vi "PopulateTreeSumary.vi"(8 "error in":errorcluster, 10 "array":T1[](array[typedef]), 11 "tree ref in":refnum<vi>) -> (0 "error out":errorcluster)   [LabVIEW 2013, in "NISE_CEF_TreeControl.lvlib"]
doc: "This VI will populate the tree control with the summary from the nodes. Use this when adding new nodes to tree"
uses:
  NISE_CEF_TreeControl.lvlib
  Node/Summary.ctl
  Node/NISE_CEF_Node.lvclass
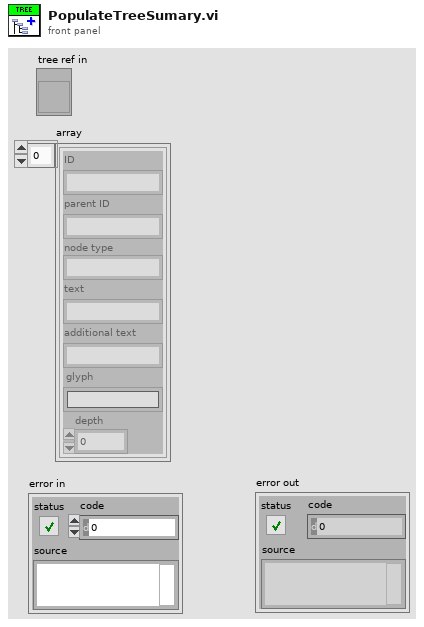
[diagram p1: front panel]
types:
  T1 = typedef "NISE_CEF_Node.lvclass/Summary.ctl" = cluster{"ID":string, "parent ID":string, "node type":string, "text":string, "additional text":string, "glyph":string, "depth":i32}
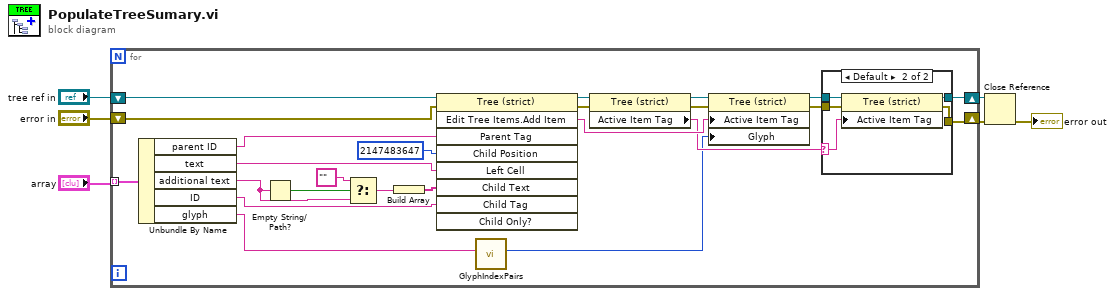
[diagram p0: block diagram]
diagram:
  n1 = for {
    tunnel: "array" -> [w15] mode=indexing
    shift-right: [w11] -> w5
    shift-left: "tree ref in" -> [w14]
    shift-right: [w9] -> w2
    shift-left: "error in" -> [w10]
    n2 = Unbundle By Name(w15) -> ("parent ID"=w30:string, "text"=w16:string, "additional text"=w8:string, "ID"=w27:string, "glyph"=w13:string)
    n3 = Empty String/Path?(string/path=w8) -> (empty?=w7:bool)
    n4 = Select(t="", s=w7, f=w8) -> (s? t:f=w25:string)
    n5 = Build Array(w25) -> (w28:string[])
    n6 = invoke class="Tree (strict)" method="Edit Tree Items.Add Item"(reference=w14, error in=w10, "Parent Tag"=w30, "Child Position"=2147483647 ("child Position"), "Left Cell"=w16, "Child Text"=w28, "Child Tag"=w27) -> (reference out=w24:refnum<vi>, error out=w23:errorcluster, "Edit Tree Items:Add Item"=w20:string)  [unwired: 2 in, 6 out]
    n7 = call "GlyphIndexPairs.vi"("glyph"=w13) -> ("index"=w12:i32)  [unwired: 10 in]
    n8 = property class="Tree (strict)"(reference=w24, error in=w23) -> (reference out=w22:refnum<vi>, error out=w21:errorcluster, "Active Item Tag"=w17:string)
    n9 = property class="Tree (strict)"(reference=w22, error in=w21, "Active Item Tag"=w20, "Glyph"=w12) -> (reference out=w19:refnum<vi>, error out=w18:errorcluster)
    n10 = case shown="Default" w17 {
      selector: w17 -> [_ w35]
      tunnel: w19 -> [w32 w37]
      tunnel: w18 -> [w31 w36]
      tunnel: [w32 w34] -> w11
      tunnel: [w31 w33] -> w9
      frame "" {
      }
      frame Default {
        n11 = property class="Tree (strict)"(reference=w37, error in=w36, "Active Item Tag"=w35) -> (reference out=w34:refnum<vi>, error out=w33:errorcluster)
      }
    }
  }
  n12 = Close Reference(reference=w5, error in (no error)=w2) -> (error out=→"error out":errorcluster)
